vi "Get FPGA Data - ECAT.vi"(8 "error in (no error)":errorcluster, 11 "Item Ref in":T1 format="%.0x") -> (0 "error out":errorcluster, 2 "FPGA":T2 {"UDVs"."To FPGA"."VS ref" format="%.0x"; "UDVs"."From FPGA"."VS ref" format="%.0x"; "VS ref" format="%.0x"; "Output Data"."BD Refs"."Data Reference" format="%.0x"; "Input Data"."BD Refs"."Data Reference" format="%.0x"}, 3 "Item Ref out":T1 format="%.0x")   [LabVIEW 2019, in "SEECD Engine.lvlib"]
uses:
  SEECD Engine.lvlib
  Type Defs/FPGA Data.ctl
  <vilib>/NI VeriStand/Custom Device API/Custom Device Item Ref.ctl
  Type Defs/Input Data.ctl
  <vilib>/NI VeriStand/Custom Device API/Block Data Reference.ctl
  <vilib>/NI VeriStand/Custom Device API/Data Reference.ctl
  Type Defs/Output Data.ctl
  Type Defs/UDV Data.ctl
  Type Defs/UDV Data Type.ctl
  Type Defs/FXP Config.ctl
  Shared/Globals/Property Strings.vi
  <vilib>/NI VeriStand/Custom Device API/Get Item Property (U32).vi
  <vilib>/NI VeriStand/Custom Device API/Custom Device API.lvlib
  Shared/SEECD Shared.lvlib
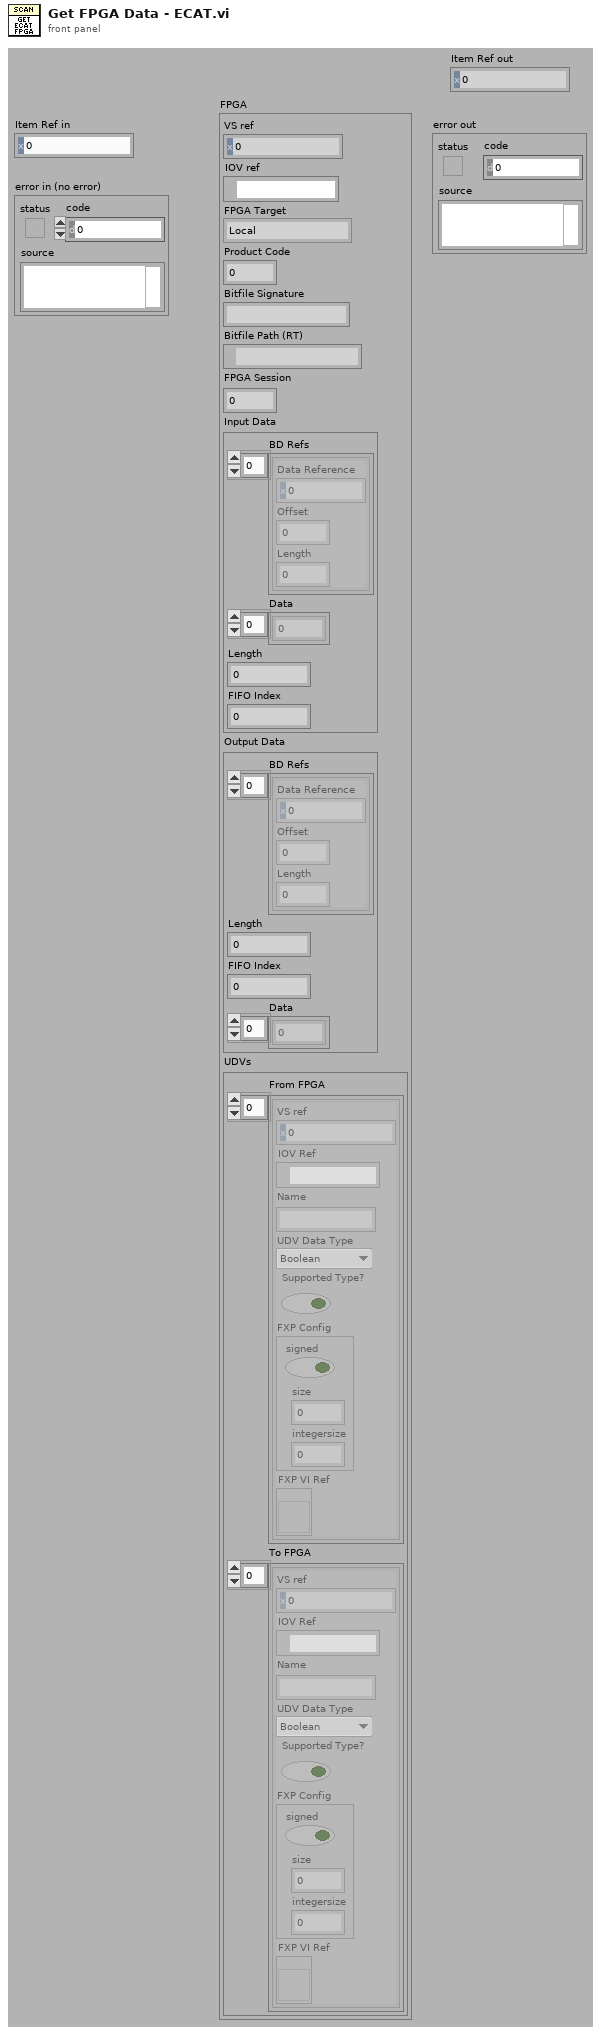
[diagram p1: front panel]
types:
  T1 = typedef "Custom Device API.lvlib/Custom Device Item Ref.ctl" = u64
  T2 = typedef "SEECD Engine.lvlib/FPGA Data.ctl" = cluster{"VS ref":T1, "IOV ref":refnum<k21>, "FPGA Target":enum16{"Local", "EtherCAT"}, "Product Code":u32, "Bitfile Signature":string, "Bitfile Path (RT)":path, "FPGA Session":u32, "Input Data":T3, "Output Data":T6, "UDVs":cluster{"From FPGA":T7[], "To FPGA":T7[]}}
  T3 = typedef "SEECD Engine.lvlib/Input Data.ctl" = cluster{"BD Refs":T4[], "Data":dbl[], "Length":i32, "FIFO Index":i32}
  T4 = typedef "Custom Device API.lvlib/Block Data Reference.ctl" = cluster{"Data Reference":T5, "Offset":u64, "Length":u64}
  T5 = typedef "Custom Device API.lvlib/Data Reference.ctl" = i32
  T6 = typedef "SEECD Engine.lvlib/Output Data.ctl" = cluster{"BD Refs":T4[], "Length":i32, "FIFO Index":i32, "Data":dbl[]}
  T7 = typedef "SEECD Engine.lvlib/UDV Data.ctl" = cluster{"VS ref":T1, "IOV Ref":refnum<k21>, "Name":string, "UDV Data Type":T8, "Supported Type?":bool, "FXP Config":T9, "FXP VI Ref":refnum<vi>}
  T8 = typedef "SEECD Engine.lvlib/UDV Data Type.ctl" = enum16{"Boolean", "Fixed Point", "Int8", "Int16", "Int32", "Int64", "U32 Bit Field", "UInt8", "UInt16", "UInt32", "UInt64", "Other", "DBL", "SGL"}
  T9 = typedef "SEECD Engine.lvlib/FXP Config.ctl" = cluster{"signed":bool, "size":u32, "integersize":i32}
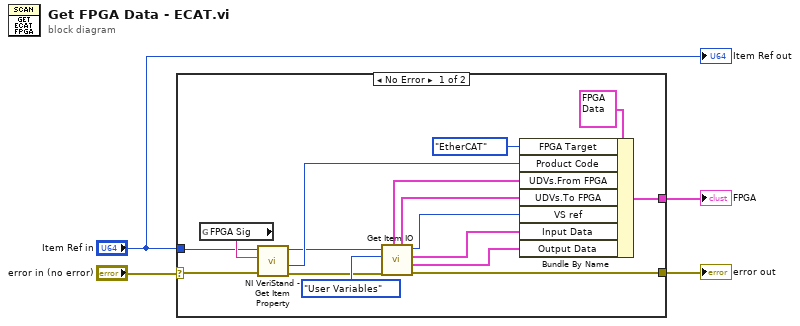
[diagram p0: block diagram]
diagram:
  n1 = case shown="No Error" "error in (no error)" {
    selector: "error in (no error)" -> [w5 w21]
    tunnel: [w20 _] -> w4
    tunnel: [w15 w21] -> w3
    tunnel: "Item Ref in" -> [w6 _]
    frame No Error {
      n2 = global read "Property Strings.vi" "FPGA Sig"() -> (w12:string)
      n3 = call-poly <vilib>:"NI VeriStand - Get Item Property.vi"("error in (no error)"=w5, "Property Name"=w12, "Item Ref in"=w6) -> ("error out"=w8:errorcluster, "Value"=w16:u32, "Item Ref out"=w7:T1)  [unwired: 5 in, 1 out]
      n4 = call "Get Item IO.vi"("error in (no error)"=w8, "Item Type"=enum16{"RSI Module", "User Variables"}."User Variables", "Item Ref in"=w7) -> ("error out"=w15:errorcluster, "Output Data"=w13:T6, "Input Data"=w14:T3, "Item Ref out"=w17:T1, "To FPGA"=w9:T7[], "From FPGA"=w10:T7[])  [unwired: 2 in, 1 out]
      n5 = Bundle By Name(cluster=T2 {"VS ref"=0, "IOV ref"="", "FPGA Target"=enum."Local", "Product Code"=0, "Bitfile Signature"="", "Bitfile Path (RT)"=path "", "FPGA Session"=0, "Input Data"={"BD Refs"=[], "Data"=[], "Length"=0, "FIFO Index"=0}, "Output Data"={"BD Refs"=[], "Length"=0, "FIFO Index"=0, "Data"=[]}, "UDVs"={"From FPGA"=[], "To FPGA"=[]}} ("FPGA"), "FPGA Target"=enum16{"Local", "EtherCAT"}."EtherCAT", "Product Code"=w16, "UDVs.From FPGA"=w10, "UDVs.To FPGA"=w9, "VS ref"=w17, "Input Data"=w14, "Output Data"=w13) -> (w20:T2)
    }
    frame Error {
    }
  }
  "FPGA" <- w4
  "error out" <- w3
  "Item Ref out" <- "Item Ref in"
